vi "Get Best Parameters.vi"(8 "error in (no error)":errorcluster, 11 "Run Optimiser in":refnum<class "Optimiser Cell.lvclass">) -> (0 "error out":errorcluster, 2 "Best Parameters":string[][](array[string]), 3 "Run Optimiser out":refnum<class "Optimiser Cell.lvclass">)   [LabVIEW 2020, in "TALOS.lvlib" / "Run Utilities.lvlib" / "Optimiser Cell.lvclass"]
uses:
  Optimiser Cell.lvclass
  Optimiser Cell.lvclass/Optimiser Cell.ctl
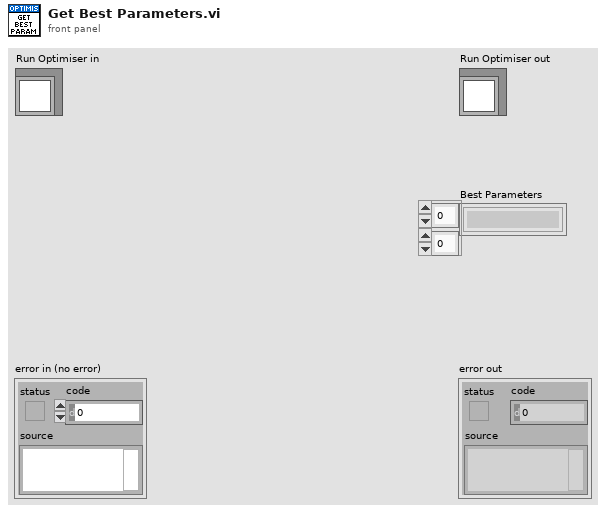
[diagram p1: front panel]
types:
  T1 = typedef "TALOS.lvlib/Run Utilities.lvlib/Optimiser Cell.lvclass/Optimiser Results.ctl" = cluster{"Array of Parameters":T2[], "Target":string}
  T2 = typedef "TALOS.lvlib/Run Utilities.lvlib/Analysis Framework.lvclass/Name with value pair.ctl" = cluster{"Name":string, "Value":string}
  T3 = typedef "TALOS.lvlib/Run Utilities.lvlib/Optimiser Cell.lvclass/Optimisation Strategy.ctl" = enum16{"Maximize", "Minimize", "Value"}
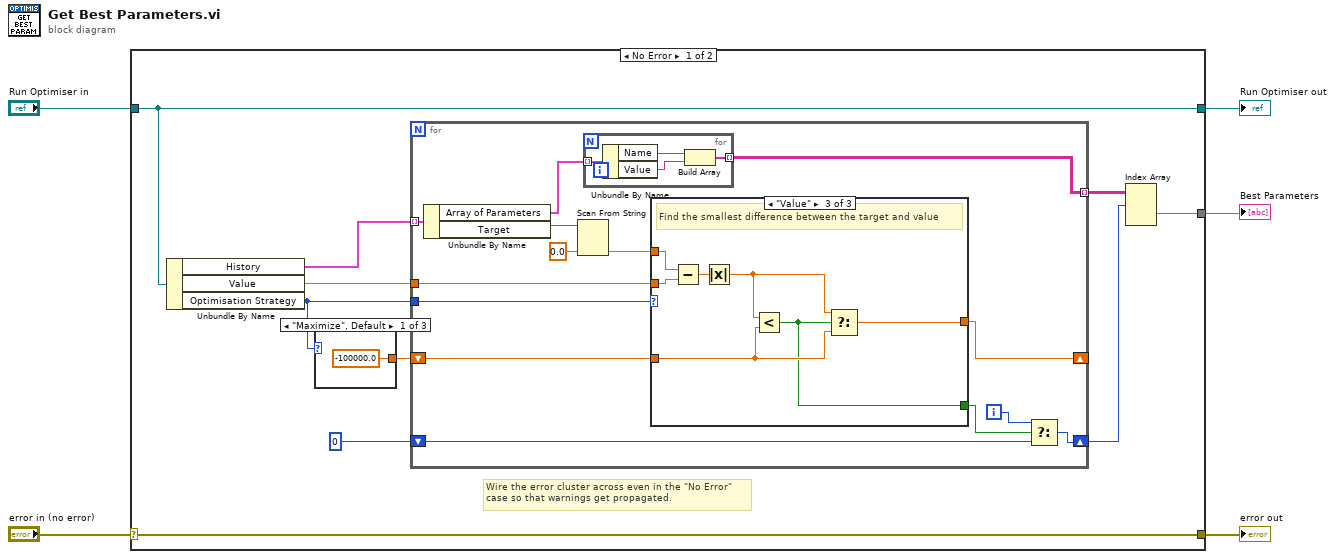
[diagram p0: block diagram]
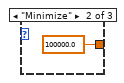
[diagram p2: hidden frame]
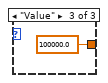
[diagram p3: hidden frame]
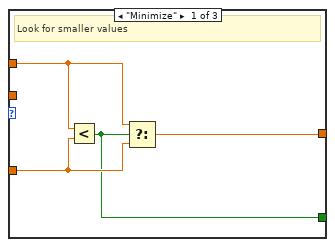
[diagram p4: hidden frame]
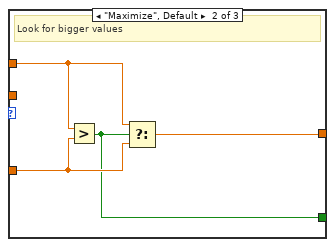
[diagram p5: hidden frame]
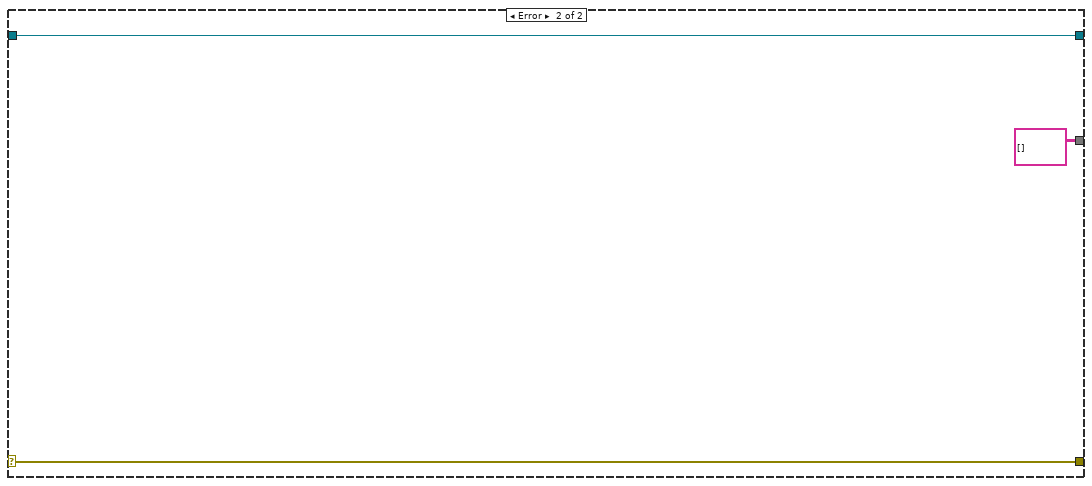
[diagram p6: hidden frame]
diagram:
  n1 = case shown="No Error" "error in (no error)" {
    selector: "error in (no error)" -> [w15 w54]
    tunnel: [w15 w54] -> w4
    tunnel: [w14 w53] -> w2
    tunnel: "Run Optimiser in" -> [w14 w53]
    tunnel: [w7 string[][] []] -> w1
    frame No Error {
      # "Wire the error cluster across even in the \"No Error\"\ncase so that warnings get propagated."
      n2 = Unbundle By Name(w14) -> ("History"=w13:T1[], "Value"=w9:dbl, "Optimisation Strategy"=w6:T3)
      n3 = case shown="\"Maximize\", Default" w6 {
        tunnel: [-100000.0 100000.0 100000.0] -> w8
        frame "Maximize", Default {
        }
        frame "Minimize" {
        }
        frame "Value" {
        }
      }
      n4 = for {
        tunnel: w13 -> [w32] mode=indexing
        tunnel: [w19] -> w11 mode=indexing
        shift-right: [w29] -> w10
        shift-left: 0 -> [w30]
        tunnel: w6 -> [w27]
        tunnel: w9 -> [w26]
        shift-right: [w21] -> _
        shift-left: w8 -> [w23]
        i -> [w31]
        n5 = Unbundle By Name(w32) -> ("Array of Parameters"=w20:T2[], "Target"=w28:string)
        n6 = Scan From String(input string=w28, default 1=0.0 ("input 1")) -> (output 1=w24:dbl)  [unwired: 3 in, 3 out]
        n7 = for {
          tunnel: w20 -> [w36] mode=indexing
          tunnel: [w33] -> w19 mode=indexing
          n8 = Unbundle By Name(w36) -> ("Name"=w35:string, "Value"=w34:string)
          n9 = Build Array(w35, w34) -> (w33:string[])
        }
        n10 = case shown="\"Value\"" w27 {
          tunnel: w26 -> [_ _ w50]
          tunnel: w24 -> [w40 w44 w51]
          tunnel: w23 -> [w39 w43 w47]
          tunnel: [w38 w42 w46] -> w21
          tunnel: [w37 w41 w45] -> w22
          frame "Minimize" {
            # "Look for smaller values"
            n11 = Less?(x=w40, y=w39) -> (x < y?=w37:bool)
            n12 = Select(t=w40, s=w37, f=w39) -> (s? t:f=w38:dbl)
          }
          frame "Maximize", Default {
            # "Look for bigger values"
            n13 = Greater?(x=w44, y=w43) -> (0:w41:bool)
            n14 = Select(t=w44, s=w41, f=w43) -> (s? t:f=w42:dbl)
          }
          frame "Value" {
            # "Find the smallest difference between the target and value"
            n15 = Subtract(x=w51, y=w50) -> (x-y=w49:dbl)
            n16 = Absolute Value(x=w49) -> (abs(x)=w48:dbl)
            n17 = Less?(x=w48, y=w47) -> (x < y?=w45:bool)
            n18 = Select(t=w48, s=w45, f=w47) -> (s? t:f=w46:dbl)
          }
        }
        n19 = Select(t=w31, s=w22, f=w30) -> (s? t:f=w29:i32)
      }
      n20 = Index Array(array=w11, index (dim 0)=w10) -> (element=w7:string[][])  [unwired: 2 in]
    }
    frame Error {
    }
  }
  "error out" <- w4
  "Run Optimiser out" <- w2
  "Best Parameters" <- w1
